vi "start_DLP_repetitions.vi"(8 "error in (no error)":errorcluster, 10 "SequenceId":u32, 11 "DeviceId":u32) -> (0 "error out":errorcluster, 2 "SequenceId Out":u32, 3 "DeviceId Out":u32)   [LabVIEW 2020]
uses:
  <vilib>/Utility/error.llb/Error Cluster From Error Code.vi
  <userlib>/alp4395/alp4395.dll
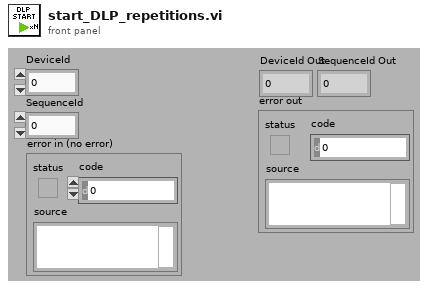
[diagram p1: front panel]
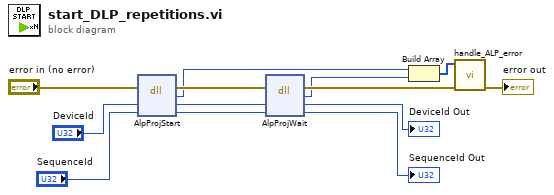
[diagram p0: block diagram]
diagram:
  n1 = dll-call lib="C:/Program Files (x86)/National Instruments/LabVIEW 2020/user.lib/alp4395/alp4395.dll" fn="AlpProjStart"(error in="error in (no error)", "DeviceId"="DeviceId", "SequenceId"="SequenceId") -> (error out=w8:errorcluster, "return type"=w6:i32, "DeviceId"=w4:u32, "SequenceId"=w3:u32)  [unwired: 2 in, 1 out]
  n2 = dll-call lib="C:/Program Files (x86)/National Instruments/LabVIEW 2020/user.lib/alp4395/alp4395.dll" fn="AlpProjWait"(error in=w8, "DeviceId"=w4, "SequenceId"=w3) -> (error out=w7:errorcluster, "return type"=w5:i32, "DeviceId"=→"DeviceId Out":u32, "SequenceId"=→"SequenceId Out":u32)  [unwired: 2 in, 1 out]
  n3 = Build Array(w6, w5) -> (w13:i32[])
  n4 = call "handle_ALP_error.vi"("error in"=w7, "Return Codes"=w13) -> ("error out"=→"error out":errorcluster)  [unwired: 9 in]
